vi "Get EM Advanced.vi"(11 "state":i32) -> (2 "function return":u32, 3 "state out":i32)   [LabVIEW 2018, in "AndorSDK.lvlib"]
doc: "EXPNETTYPE unsigned int WINAPI GetEMAdvanced(int * state);"
uses:
  AndorSDK.lvlib
  ATMCD32D.dll
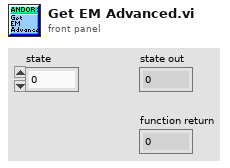
[diagram p1: front panel]
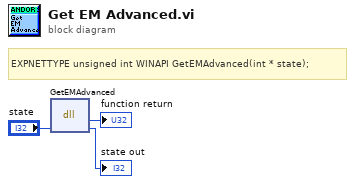
[diagram p0: block diagram]
diagram:
  # "EXPNETTYPE unsigned int WINAPI GetEMAdvanced(int * state);"
  n1 = dll-call lib="PTH2babs E\nPersönliches02 - Arbeit03-HiwijobsLabviewCodelibANDOR\tAndor SDK\nATMCD32D.*" fn="GetEMAdvanced"("state"="state") -> (→"function return":u32, "state"=→"state out":i32)  [unwired: 3 in, 2 out]
